vi "CCD_Initialization V0.49.vi"(6 "error in":errorcluster, 7 "Setup String":string="ldb,1,16,u,0,225,25,b,1,15;sdu,0,1024,1024;cl0;omrm;sron", 8 "CCD GPIB Address":u8=1 min=1 max=1) -> (0 "error out":errorcluster, 2 "Error (0=No Error)":i16=-1, 3 "Poll Status":bool[](array[boolean])=[FALSE, FALSE, TRUE, FALSE, TRUE, TRUE, TRUE, FALSE, TRUE, FALSE, FALSE, FALSE, FALSE, FALSE, FALSE, FALSE], 5 "Poll Byte":i16)   [LabVIEW 2021]
doc: "Resets the CCD camera controller and initializes it with Setup String. The default Setup String is \"ldb,1,16,u,0,225,25,b,1,15;sdu,0,1024,1024;cl0;omrm;sron\". \nError, if no -1, is set as 0 if a serial poll detects an error (bit 15 in status bit set)\n\nSet the CCD Setup String Global variable after the command is complete."
uses:
  Globals and TypeDefs/Global Varibal Control.vi
panel:
  out "Setup String sent":string="ldu,0,256,16;sdu,0,1024,1024;cl0;omrm;sron"
  out "SRQWait error out":errorcluster
  out "GPIB SRQ status output":bool[](array[boolean])
  out "SRQ":bool
  out "SetupTime (s)":dbl=2.799 format="%.2f"
  out "Current Action":u16(ring) items=["InitializeGPIB", "Poll CCD Controller", "Wait for CCD SRQ", "Setup CCD Camera", "Wait for CCD SRQ-S"]
  out "Poll StatusNo":u16=372
  out "GPIB Error":u16
  # "Status Byte:\n[0]: Dev.Clear State  [8]: Oper.Complete\n[1]: Dev.Trig.State    [9]:   ---\n[2]: Listener Active   [10]: ---\n[3]: Talker Active      [11]: ---\n[4]: Attn. Asserted    [12]: SRQ det.whl CIC\n[5]: CIC                      [13]: EOI or EOS det.\n[6]: Remote State       [14]: Timeout\n[7]: Lockout State       [15]: Error detected"
  # "15"
  # "Initial Errors..."
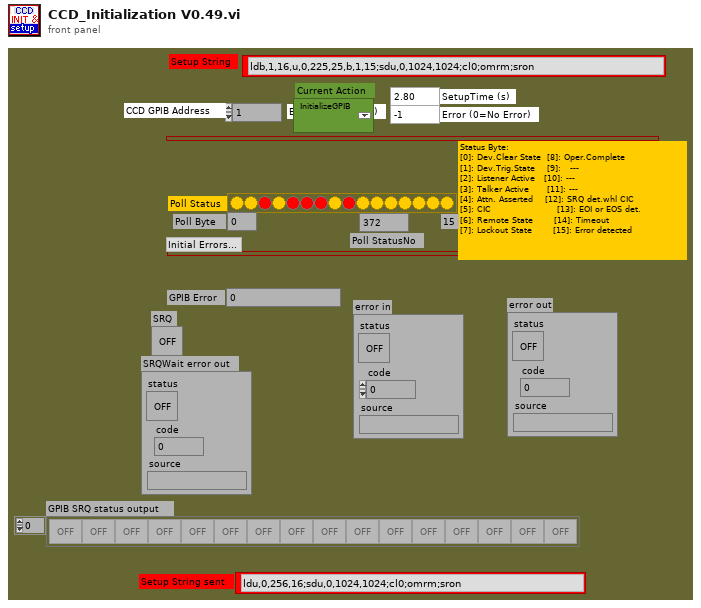
[diagram p1: front panel]
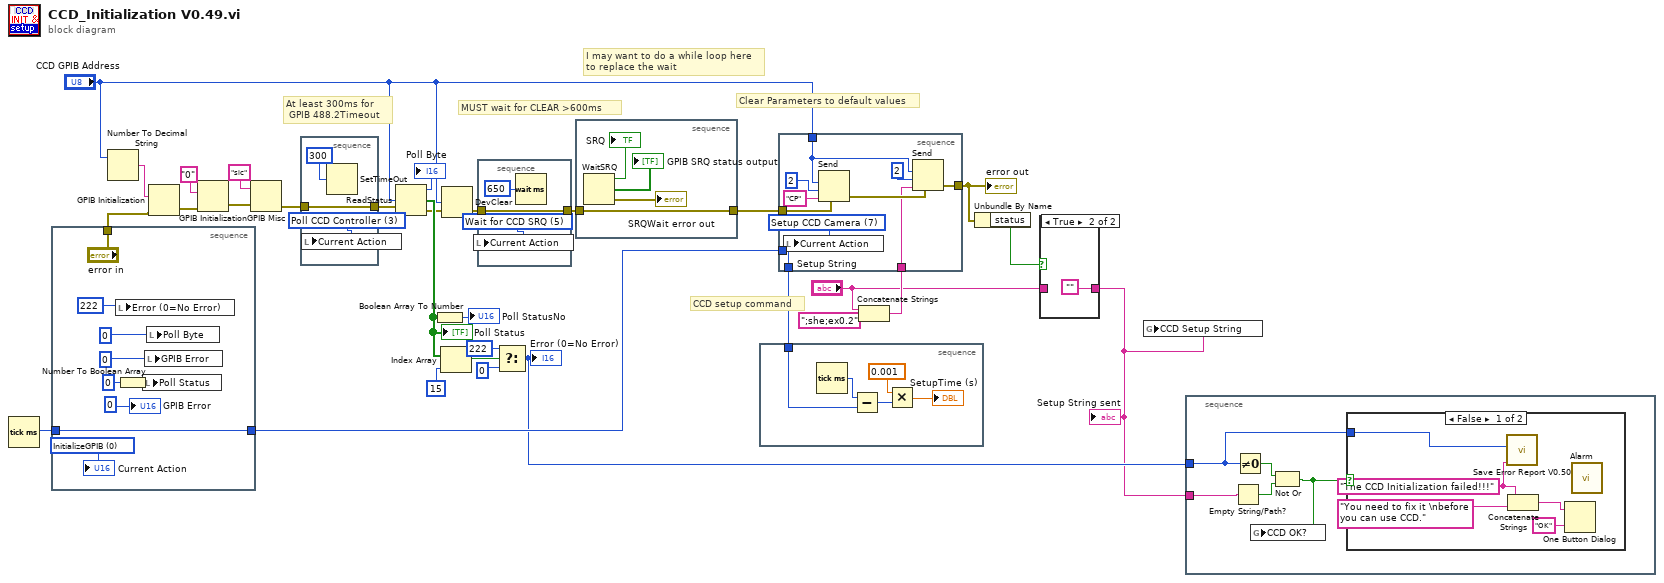
[diagram p0: block diagram]
diagram:
  # "I may want to do a while loop here\nto replace the wait"
  # "CCD setup command"
  # "Clear Parameters to default values"
  # "MUST wait for CLEAR >600ms"
  # "At least 300ms for \n GPIB 488.2Timeout"
  n1 = Tick Count (ms)() -> (millisecond timer value=w19:u32)
  n2 = stacked-sequence {
    tunnel: w19 -> [w33]
    tunnel: [w33] -> w17
    tunnel: ["error in"] -> w14
    frame #0 {
      w32 = u16 0 items=["InitializeGPIB", "GPIB Bus Scan", "Get CCD Status", "Poll CCD Controller", "Clear CCD Controller", "Wait for CCD SRQ", "Clear CCD Parms.", "Setup CCD Camera", "Take Dark Spectrum", "Wait for CCD SRQ-S", "Read out Dark Data", "Enable Shutter"] ("Current Action")
      n3 = local write "Error (0=No Error)"(i16 222) -> ()
      n4 = Number To Boolean Array(number=u16 0) -> (Boolean array=w36:bool[])
      n5 = local write "Poll Status"(w36) -> ()
      n6 = local write "GPIB Error"(u16 0) -> ()
      n7 = local write "Poll Byte"(i16 0) -> ()
      "GPIB Error" <- u16 0
      "Current Action" <- w32
    }
  }
  n8 = Number To Decimal String(number="CCD GPIB Address") -> (decimal integer string=w9:string)  [unwired: 1 in]
  n9 = GPIB Initialization(4:w14, 6:w9) -> (0:w13:errorcluster)  [unwired: 5 in]
  n10 = GPIB Initialization(4:w13, 6:"0" ("address string")) -> (0:w12:errorcluster)  [unwired: 5 in]
  n11 = GPIB Misc(0:"sic", 1:w12) -> (4:w11:errorcluster)  [unwired: 2 out]
  n12 = stacked-sequence {
    tunnel: w11 -> [w41]
    tunnel: [w41] -> w20
    frame #0 {
      w40 = u16 3 items=["InitializeGPIB", "GPIB Bus Scan", "Get CCD Status", "Poll CCD Controller", "Clear CCD Controller", "Wait for CCD SRQ", "Clear CCD Parms.", "Setup CCD Camera", "Take Dark Spectrum", "Wait for CCD SRQ-S", "Read out Dark Data", "Enable Shutter"] ("Current Action")
      n13 = local write "Current Action"(w40) -> ()
      n14 = SetTimeOut(1:300 ("new timeout (10000)")) -> ()  [unwired: 1 out]
    }
  }
  n15 = ReadStatus(3:w20, 4:"CCD GPIB Address") -> (0:w23:errorcluster, 1:w30:bool[], 2:→"Poll Byte":i16)  [unwired: 1 in]
  "Poll Status" <- w30
  n16 = Boolean Array To Number(Boolean array=w30) -> (number=→"Poll StatusNo":u32)
  n17 = Index Array(array=w30, index=15) -> (element=w28:bool)
  n18 = DevClear(2:w23, 3:"CCD GPIB Address") -> (0:w22:errorcluster)  [unwired: 1 in, 1 out]
  n19 = stacked-sequence {
    tunnel: w22 -> [w44]
    tunnel: [w44] -> w7
    frame #0 {
      w43 = u16 5 items=["InitializeGPIB", "GPIB Bus Scan", "Get CCD Status", "Poll CCD Controller", "Clear CCD Controller", "Wait for CCD SRQ", "Clear CCD Parms.", "Setup CCD Camera", "Take Dark Spectrum", "Wait for CCD SRQ-S", "Read out Dark Data", "Enable Shutter"] ("Current Action")
      n20 = local write "Current Action"(w43) -> ()
      n21 = Wait (ms)(milliseconds to wait=u32 650) -> ()  [unwired: 1 out]
    }
  }
  n22 = Select(t=i16 222, s=w28, f=i16 0) -> (s? t:f=w2:i16)
  "Error (0=No Error)" <- w2
  n23 = stacked-sequence {
    tunnel: [w49] -> w6
    tunnel: w7 -> [w49]
    frame #0 {
      n24 = WaitSRQ() -> (2:→"SRQ":bool, 3:→"GPIB SRQ status output":bool[], 4:→"SRQWait error out":errorcluster)  [unwired: 2 in]
    }
  }
  n25 = Concatenate Strings("Setup String", ";she;ex0.2") -> (w18:string)
  n26 = stacked-sequence {
    tunnel: w6 -> [w57]
    tunnel: "CCD GPIB Address" -> [w54]
    tunnel: w18 -> [w52]
    tunnel: [w51] -> w5
    tunnel: w17 -> [w50]
    tunnel: [w50] -> w16
    frame #0 {
      w53 = u16 7 items=["InitializeGPIB", "GPIB Bus Scan", "Get CCD Status", "Poll CCD Controller", "Clear CCD Controller", "Wait for CCD SRQ", "Clear CCD Parms.", "Setup CCD Camera", "Take Dark Spectrum", "Wait for CCD SRQ-S", "Read out Dark Data", "Enable Shutter"] ("Current Action")
      n27 = local write "Current Action"(w53) -> ()
      n28 = Send(2:w54, 3:u8 2, 4:w57, 5:"CP") -> (8:w55:errorcluster)  [unwired: 1 in, 2 out]
      n29 = Send(2:w54, 3:u8 2, 4:w55, 5:w52) -> (8:w51:errorcluster)  [unwired: 1 in, 2 out]
    }
  }
  "error out" <- w5
  n30 = stacked-sequence {
    tunnel: w16 -> [w60]
    frame #0 {
      n31 = Tick Count (ms)() -> (millisecond timer value=w61:u32)
      n32 = Subtract(x=w61, y=w60) -> (x-y=w62:u32)
      n33 = Multiply(x=0.001, y=w62) -> (x*y=→"SetupTime (s)":dbl)
    }
  }
  n34 = Unbundle By Name(w5) -> ("status"=w4:bool)
  n35 = case shown="True" w4 {
    tunnel: [w65 ""] -> w1
    tunnel: "Setup String" -> [w65 _]
    frame False {
    }
    frame True {
    }
  }
  "Setup String sent" <- w1
  n36 = global write "Global Varibal Control.vi" "CCD Setup String"(w1) -> ()
  n37 = stacked-sequence {
    tunnel: w2 -> [w69]
    tunnel: w1 -> [w68]
    frame #0 {
      n38 = Empty String/Path?(string/path=w68) -> (empty?=w70:bool)
      n39 = Not Equal To 0?(x=w69) -> (x != 0?=w71:bool)
      n40 = Not Or(1:w70, 2:w71) -> (0:w67:bool)
      n41 = global write "Global Varibal Control.vi" "CCD OK?"(w67) -> ()
      n42 = case shown="False" w67 {
        tunnel: w69 -> [w72 _]
        frame False {
          w73 = "The CCD Initialization failed!!!" ("message")
          n43 = call "Save Error Report V0.50.vi"("Error Message"=w73, "Error Code (0: No Error)"=w72) -> ()  [unwired: 4 in, 1 out]
          n44 = Concatenate Strings(w73, "You need to fix it \nbefore you can use CCD." ("message")) -> (w74:string)
          n45 = One Button Dialog(message=w74, button name ("OK")="OK") -> ()  [unwired: 1 out]
          n46 = call "Alarm.vi"() -> ()  [unwired: 4 in]
        }
        frame True {
        }
      }
    }
  }
